vi "addHoneycomb.vi"() -> ()   [LabVIEW 2015]
uses:
  GlobalPath.vi
  GlobalData.vi
  GlobalVi.vi
panel:
  in  "Done?":bool
  in  "HONEYCOMB 4":string
  in  "HONEYCOMB 3":string
  in  "HONEYCOMB 2":string
  in  "ptfe 2":bool caption="Position the honeycomb on top of each PCB on the table"
  in  "Save the IDs in the database?":bool
  in  "Fill database with honeycomb IDs?\nTo do so go to the database, select the Honeycomb tab, choose the correct frame ID and press \"check_db\"\nThen click on \"Add/Update Entry\"":bool
  in  "HONEYCOMB 1":string
  in  "HONEYCOMB 5":string
  # "Add honeycomb"
  # "Adding the honeycomb ID to the database"
  # "Save the ID of each of the 5 honeycomb pieces and associate them with the panel"
  # "Honeycomb ID recording"
  # "Fill each box with the ID of each honeycomb part and press SAVE"
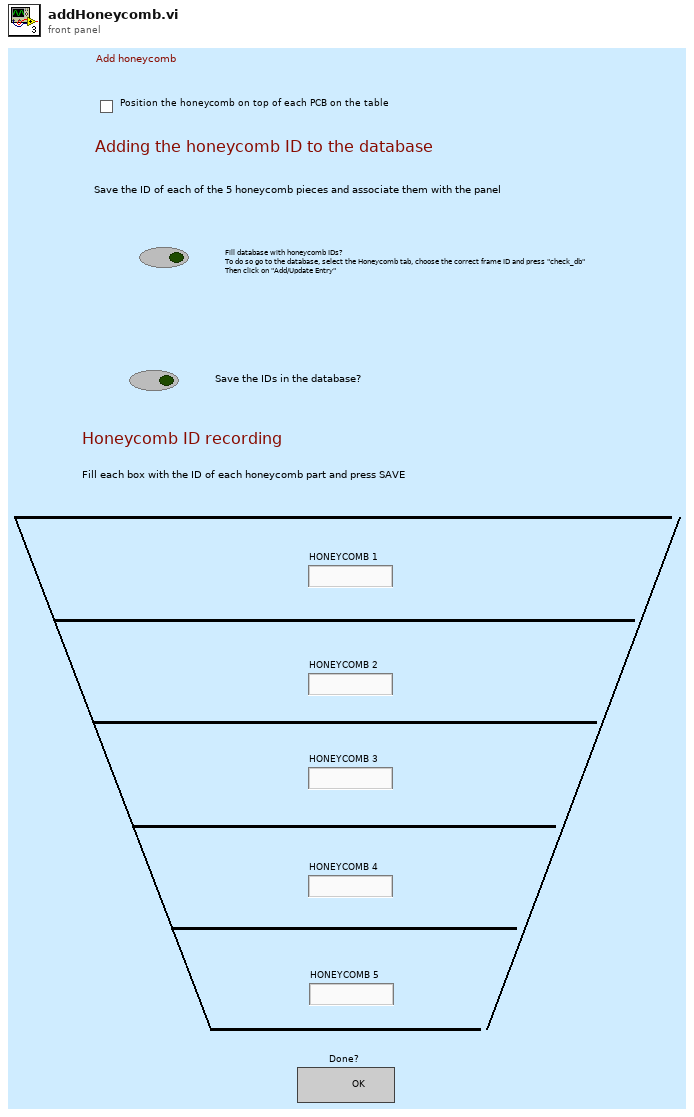
[diagram p1: front panel]
types:
  T1 = enum16{"open", "replace", "create", "open or create", "replace or create", "replace or create with confirmation"}
  T2 = enum32{"Bad", "Idle", "Run top level", "Running"}
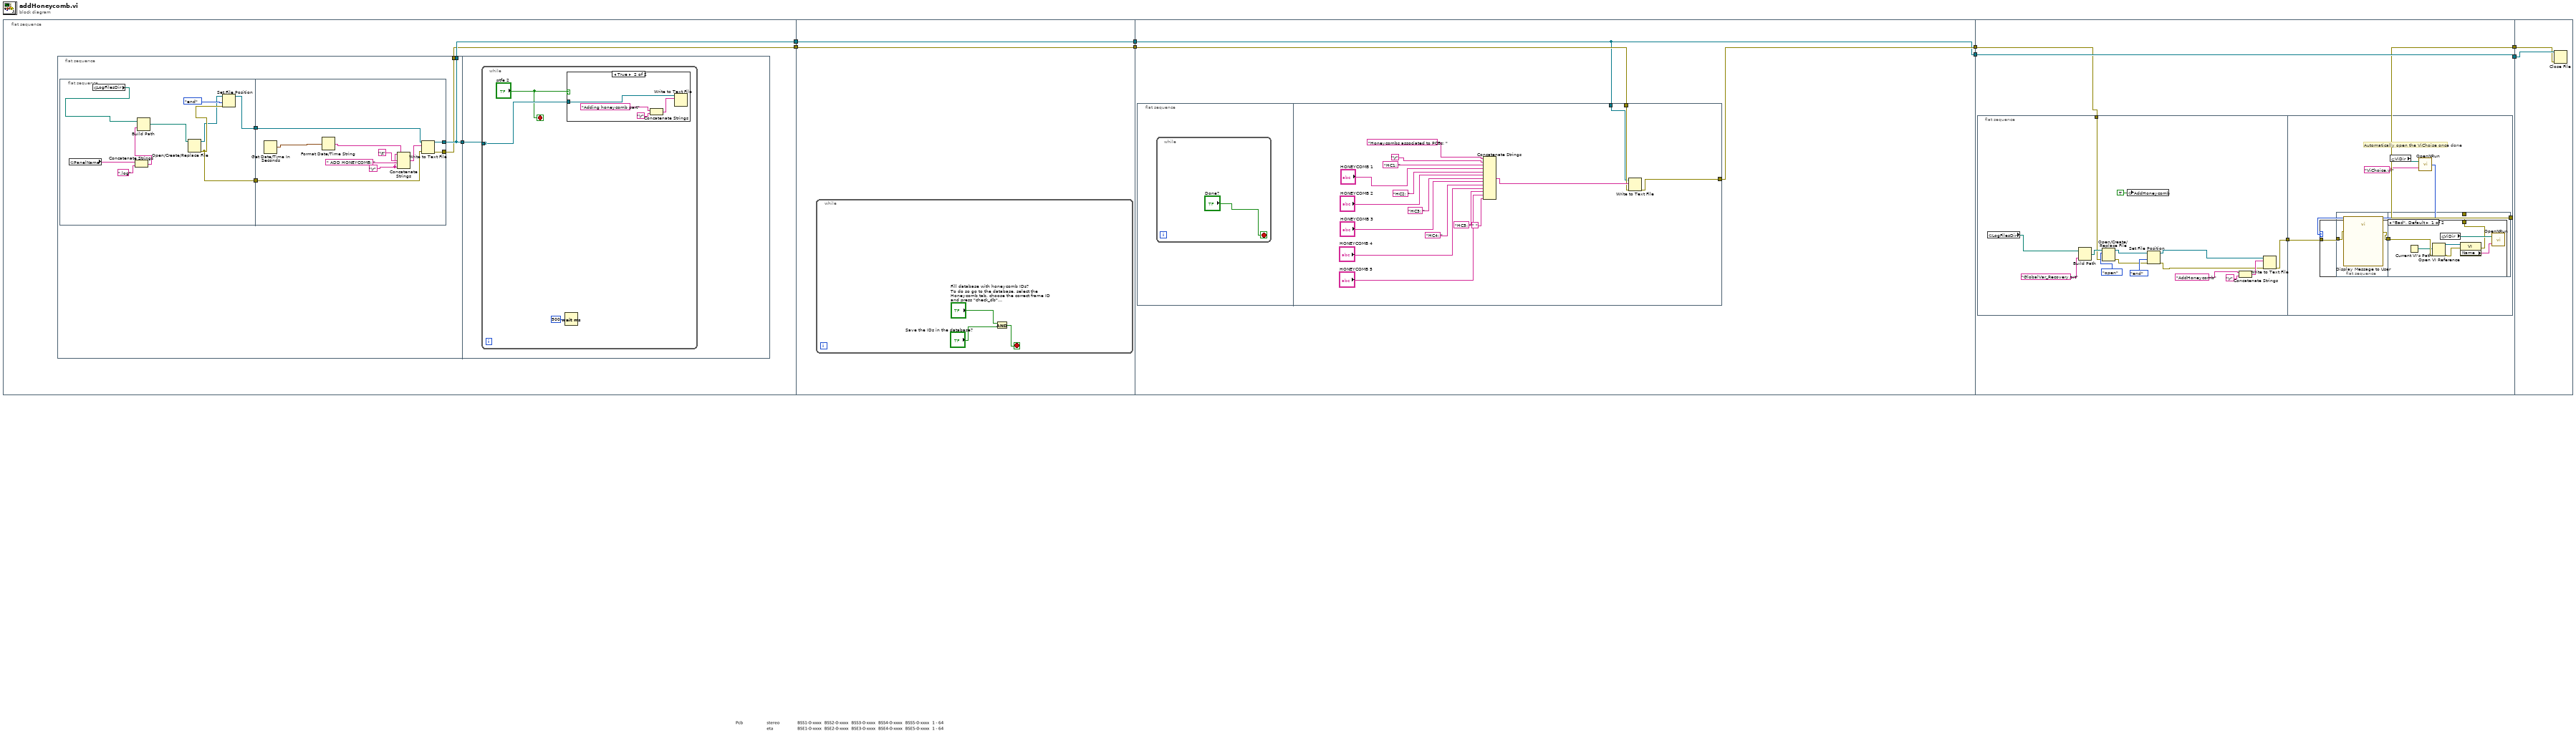
[diagram p0: block diagram]
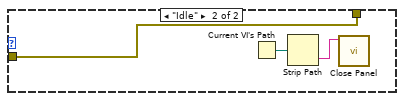
[diagram p3: hidden frame]
diagram:
  n1 = flat-sequence {
    tunnel: [w10] -> w8
    tunnel: [w9] -> w7
    tunnel: w8 -> [w44]
    tunnel: [w44] -> w2
    tunnel: w7 -> [w43]
    tunnel: [w43] -> w1
    tunnel: w2 -> [w48]
    tunnel: [w49] -> w5
    tunnel: w1 -> [w50]
    tunnel: [w48] -> w4
    tunnel: [w71] -> w6
    tunnel: w5 -> [w69]
    tunnel: w4 -> [w72]
    tunnel: [w72] -> w3
    tunnel: w6 -> [w108]
    tunnel: w3 -> [w109]
    frame #0 {
      n2 = flat-sequence {
        tunnel: [w14] -> w11
        tunnel: [w14] -> w10
        tunnel: [w13] -> w9
        tunnel: w11 -> [w35]
        frame #0 {
          n3 = flat-sequence {
            tunnel: [w17] -> w15
            tunnel: [w19] -> w12
            tunnel: w15 -> [w30]
            tunnel: [w29] -> w14
            tunnel: [w28] -> w13
            tunnel: w12 -> [w27]
            frame #0 {
              n4 = global read "GlobalData.vi" "PanelName"() -> (w23:string)
              n5 = global read "GlobalPath.vi" "LogFilesDir"() -> (w16:path)
              n6 = Concatenate Strings(w23, ".log") -> (w22:string)
              n7 = Build Path(base path=w16, name or relative path=w22) -> (appended path=w21:path)
              n8 = Open/Create/Replace File(file path (use dialog)=w21) -> (refnum out=w18:refnum<file>, error out=w19:errorcluster)  [unwired: 5 in, 1 out]
              n9 = Set File Position(refnum=w18, from (0:start)=enum16{"start", "end", "current"}."end", error in=w19) -> (refnum out=w17:refnum<file>)  [unwired: 1 in, 1 out]
            }
            frame #1 {
              w25 = "\r"
              n10 = Get Date/Time In Seconds() -> (seconds since 1Jan1904=w26:timestamp)
              n11 = Format Date/Time String(seconds (now)=w26) -> (date/time string=w32:string)  [unwired: 2 in]
              n12 = Concatenate Strings(w25, w32, "\t", " ADD HONEYCOMB: ", w25) -> (w31:string)
              n13 = Write to Text File(file (use dialog)=w30, text=w31, error in=w27) -> (refnum out=w29:refnum<file>, error out=w28:errorcluster)  [unwired: 1 in, 1 out]
            }
          }
        }
        frame #1 {
          n14 = while {
            tunnel: w35 -> [w37]
            stop <- "ptfe 2" stop-if-true
            n15 = Wait (ms)(milliseconds to wait=u32 500) -> ()  [unwired: 1 out]
            n16 = case shown="True" "ptfe 2" {
              tunnel: w37 -> [_ w39]
              frame False {
              }
              frame True {
                n17 = Concatenate Strings("Adding honeycomb part", "\r") -> (w42:string)
                n18 = Write to Text File(file (use dialog)=w39, text=w42) -> ()  [unwired: 2 in, 3 out]
              }
            }
          }
        }
      }
    }
    frame #1 {
      n19 = while {
        stop <- w45 stop-if-true
        n20 = And(x="Fill database with honeycomb IDs?\nTo do so go to the database, select the Honeycomb tab, choose the correct frame ID and press \"check_db\"\nThen click on \"Add/Update Entry\"", y="Save the IDs in the database?") -> (x .and. y?=w45:bool)
      }
    }
    frame #2 {
      n21 = flat-sequence {
        tunnel: [w64] -> w49
        tunnel: w50 -> [w63]
        tunnel: w48 -> [w62]
        frame #0 {
          n22 = while {
            stop <- "Done?" stop-if-true
          }
        }
        frame #1 {
          n23 = Concatenate Strings("Honeycombs associated to PCBs: ", "\r", "HC1: ", "HONEYCOMB 1", "HC2: ", "HONEYCOMB 2", "HC3: ", "HONEYCOMB 3", "HC4: ", "HONEYCOMB 4", "HC5: ", "HONEYCOMB 5", " ") -> (w65:string)
          n24 = Write to Text File(file (use dialog)=w62, text=w65, error in=w63) -> (error out=w64:errorcluster)  [unwired: 1 in, 2 out]
        }
      }
    }
    frame #3 {
      n25 = flat-sequence {
        tunnel: [w75] -> w70
        tunnel: w69 -> [w76]
        tunnel: [w88] -> w71
        tunnel: w70 -> [w89]
        frame #0 {
          n26 = global read "GlobalPath.vi" "LogFilesDir"() -> (w73:path)
          n27 = Build Path(base path=w73, name or relative path="GlobalVar_Recovery.txt") -> (appended path=w85:path)
          n28 = Open/Create/Replace File(file path (use dialog)=w85, error in=w76, operation (0:open)=T1."open") -> (refnum out=w81:refnum<file>, error out=w82:errorcluster)  [unwired: 3 in, 1 out]
          n29 = global write "GlobalVi.vi" "AddHoneycomb"(TRUE) -> ()
          n30 = Set File Position(refnum=w81, from (0:start)=enum16{"start", "end", "current"}."end", error in=w82) -> (refnum out=w78:refnum<file>, error out=w77:errorcluster)  [unwired: 1 in]
          n31 = Concatenate Strings("AddHoneycomb", "\r") -> (w80:string)
          n32 = Write to Text File(file (use dialog)=w78, text=w80, error in=w77) -> (error out=w75:errorcluster)  [unwired: 1 in, 2 out]
        }
        frame #1 {
          # "Automatically open the ViChoise once done"
          n33 = global read "GlobalPath.vi" "ViDir"() -> (w92:path)
          n34 = call "OpenNRun.vi"("VI name"="ViChoice.vi", "ViDirPath"=w92) -> ("Execution:State"=w91:T2)
          n35 = case shown="\"Bad\", Default" w91 {
            tunnel: [w93 w105] -> w88
            tunnel: w89 -> [w94 w105]
            frame "Bad", Default {
              n36 = flat-sequence {
                tunnel: w94 -> [w97]
                tunnel: [w96] -> w95
                tunnel: w95 -> [w101]
                tunnel: [w98] -> w93
                frame #0 {
                  n37 = call "Display Message to User"("error in (no error)"=w97) -> ("error out"=w96:errorcluster)  [unwired: 9 in, 1 out]
                }
                frame #1 {
                  n38 = Current VI's Path() -> (path=w99:path)
                  n39 = Open VI Reference(vi path=w99, error in (no error)=w101) -> (vi reference=w104:refnum<vi>, error out=w103:errorcluster)  [unwired: 4 in]
                  n40 = global read "GlobalPath.vi" "ViDir"() -> (w100:path)
                  n41 = property class="VI"(reference=w104, error in=w103) -> (error out=w98:errorcluster, "Name"=w102:string)  [unwired: 1 out]
                  n42 = call "OpenNRun.vi"("VI name"=w102, "ViDirPath"=w100) -> ()  [unwired: 1 out]
                }
              }
            }
            frame "Idle" {
              n43 = Current VI's Path() -> (path=w106:path)
              n44 = Strip Path(path=w106) -> (name=w107:string)  [unwired: 1 out]
              n45 = call <vilib>:"Close Panel.vi"("VI name"=w107) -> ()  [unwired: 10 in, 1 out]
            }
          }
        }
      }
    }
    frame #4 {
      n46 = Close File(refnum=w109, error in=w108) -> ()  [unwired: 2 out]
    }
  }
